vi "chart_clustered.vi"() -> ()   [LabVIEW 8.6]
uses:
  Controls/lxw_chart_type.ctl
  Controls/style_id.ctl
  Controls/lxw_chart_legend_position.ctl
panel:
  out "error out":errorcluster
  out "function return 2":string
  # "chart_clustered2.xlsx"
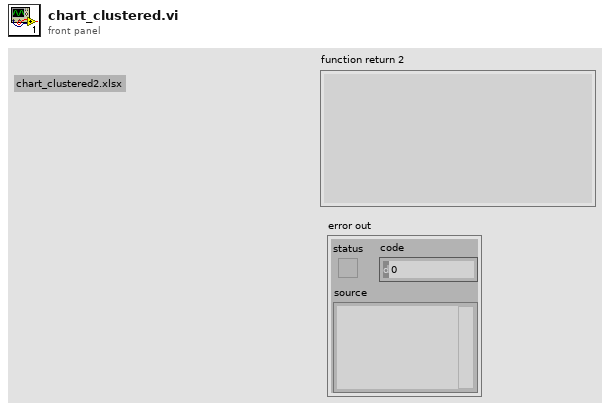
[diagram p1: front panel]
types:
  T1 = typedef "lxw_chart_legend_position.ctl" = u8
  T2 = typedef "style_id.ctl" = u16
  T3 = typedef "lxw_chart_type.ctl" = u8
  T4 = enum32{"invalid app kind", "Development System", "Run Time System", "Student Edition", "Embedded LabVIEW", "Evaluation", "Custom"}
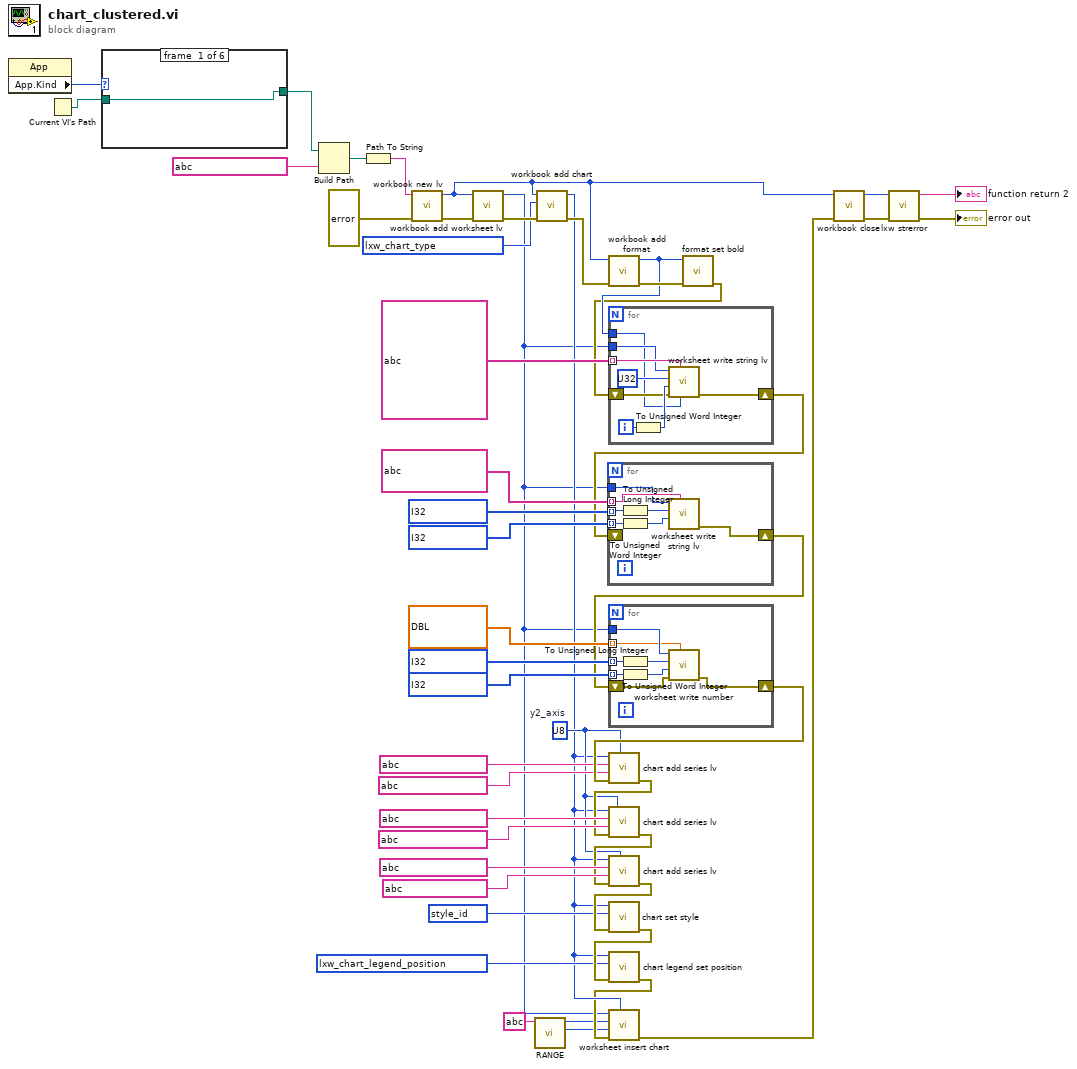
[diagram p0: block diagram]
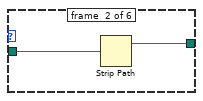
[diagram p2: hidden frame]
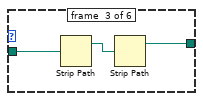
[diagram p3: hidden frame]
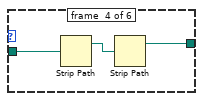
[diagram p4: hidden frame]
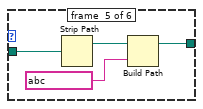
[diagram p5: hidden frame]
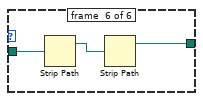
[diagram p6: hidden frame]
diagram:
  w9 = T1 ? items=["LXW_CHART_LEGEND_NONE", "LXW_CHART_LEGEND_RIGHT", "LXW_CHART_LEGEND_LEFT", "LXW_CHART_LEGEND_TOP", "LXW_CHART_LEGEND_BOTTOM", "LXW_CHART_LEGEND_TOP_RIGHT", "LXW_CHART_LEGEND_OVERLAY_RIGHT", "LXW_CHART_LEGEND_OVERLAY_LEFT", "LXW_CHART_LEGEND_OVERLAY_TOP_RIGHT"] ("position")
  w11 = T2 ? items=["Style_1", "Style_2", "Style_3", "Style_4", "Style_5", "Style_6", "Style_7", "Style_8", "Style_9", "Style_10", "Style_11", "Style_12", "Style_13", "Style_14", "Style_15", "Style_16", "Style_17", "Style_18", "Style_19", "Style_20", "Style_21", "Style_22", "Style_23", "Style_24", "Style_25", "Style_26", "Style_27", "Style_28", "Style_29", "Style_30", "Style_31", "Style_32", "Style_33", "Style_34", "Style_35", "Style_36", "Style_37", "Style_38", "Style_39", "Style_40", "Style_41", "Style_42", "Style_43", "Style_44", "Style_45", "Style_46", "Style_47", "Style_48"] ("style_id")
  w12 = u8 ?  # y2_axis
  w27 = T3 ? items=["LXW_CHART_NONE", "LXW_CHART_AREA", "LXW_CHART_AREA_STACKED", "LXW_CHART_AREA_STACKED_PERCENT", "LXW_CHART_BAR", "LXW_CHART_BAR_STACKED", "LXW_CHART_BAR_STACKED_PERCENT", "LXW_CHART_COLUMN", "LXW_CHART_COLUMN_STACKED", "LXW_CHART_COLUMN_STACKED_PERCENT", "LXW_CHART_DOUGHNUT", "LXW_CHART_LINE", "LXW_CHART_LINE_STACKED", "LXW_CHART_LINE_STACKED_PERCENT", "LXW_CHART_PIE", "LXW_CHART_SCATTER", "LXW_CHART_SCATTER_STRAIGHT", "LXW_CHART_SCATTER_STRAIGHT_WITH_MARKERS", "LXW_CHART_SCATTER_SMOOTH", "LXW_CHART_SCATTER_SMOOTH_WITH_MARKERS", "LXW_CHART_RADAR", "LXW_CHART_RADAR_WITH_MARKERS", "LXW_CHART_RADAR_FILLED", "LXW_CHART_STOCK"] ("chart_type")
  n1 = property class="App"() -> ("App.Kind"=w49:T4)  [unwired: 2 in, 2 out]
  n2 = Current VI's Path() -> (path=w48:path)
  n3 = case shown="\"Evaluation\"" w49 {
    tunnel: w48 -> [w50 w52 w55 w58 w62 w65]
    tunnel: [w50 w51 w53 w56 w60 w63] -> w47
    frame #0 {
    }
    frame #1 {
      n4 = Strip Path(path=w52) -> (stripped path=w51:path)  [unwired: 1 out]
    }
    frame #2 {
      n5 = Strip Path(path=w55) -> (stripped path=w54:path)  [unwired: 1 out]
      n6 = Strip Path(path=w54) -> (stripped path=w53:path)  [unwired: 1 out]
    }
    frame #3 {
      n7 = Strip Path(path=w58) -> (stripped path=w57:path)  [unwired: 1 out]
      n8 = Strip Path(path=w57) -> (stripped path=w56:path)  [unwired: 1 out]
    }
    frame #4 {
      n9 = Strip Path(path=w62) -> (stripped path=w61:path)  [unwired: 1 out]
      n10 = Build Path(base path=w61, name or relative path=string ?) -> (appended path=w60:path)
    }
    frame #5 {
      n11 = Strip Path(path=w65) -> (stripped path=w64:path)  [unwired: 1 out]
      n12 = Strip Path(path=w64) -> (stripped path=w63:path)  [unwired: 1 out]
    }
  }
  n13 = Build Path(base path=w47, name or relative path=string ? ("filename")) -> (appended path=w39:path)
  n14 = Path To String(path=w39) -> (string=w38:string)
  n15 = call "workbook new lv.vi"("error in (no error)"=errorcluster ?, "filename"=w38) -> ("error out"=w45:errorcluster, "function return"=w1:u32)  [unwired: 8 in]
  n16 = call "workbook add worksheet lv.vi"("error in (no error)"=w45, "workbook"=w1) -> ("error out"=w28:errorcluster, "function return"=w6:u32)  [unwired: 8 in]
  n17 = call "RANGE.vi"("range_str"=string ?) -> ("col"=w5:u16, "row"=w4:u32)  [unwired: 6 in, 3 out]
  n18 = call "workbook add chart.vi"("error in (no error)"=w28, "chart_type"=w27, "workbook"=w1) -> ("error out"=w26:errorcluster, "function return"=w8:u32)  [unwired: 7 in]
  n19 = call "workbook add format.vi"("error in (no error)"=w26, "workbook"=w1) -> ("error out"=w30:errorcluster, "function return"=w29:u32)  [unwired: 8 in]
  n20 = call "format set bold.vi"("error in (no error)"=w30, "format"=w29) -> ("error out"=w25:errorcluster)  [unwired: 9 in]
  n21 = for {
    tunnel: string[] ? -> [w73] mode=indexing
    tunnel: w6 -> [w72]
    shift-right: [w68] -> w24
    shift-left: w25 -> [w67]
    tunnel: w29 -> [w66]
    i -> [w70]
    n22 = To Unsigned Word Integer(number=w70) -> (unsigned 16bit integer=w69:u16)
    n23 = call "worksheet write string lv.vi"("format"=w66, "string"=w73, "error in (no error)"=w67, "col"=w69, "row"=u32 ?, "worksheet"=w72) -> ("error out"=w68:errorcluster)  [unwired: 4 in, 1 out]
  }
  n24 = for {
    tunnel: string[] ? -> [w80] mode=indexing
    tunnel: i32[] ? -> [w79] mode=indexing
    tunnel: i32[] ? -> [w78] mode=indexing
    tunnel: w6 -> [w77]
    shift-right: [w74] -> w23
    shift-left: w24 -> [_]
    n25 = To Unsigned Long Integer(number=w79) -> (unsigned 32bit integer=w75:u32)
    n26 = To Unsigned Word Integer(number=w78) -> (unsigned 16bit integer=w76:u16)
    n27 = call "worksheet write string lv.vi"("string"=w80, "col"=w76, "row"=w75, "worksheet"=w77) -> ("error out"=w74:errorcluster)  [unwired: 6 in, 1 out]
  }
  n28 = for {
    tunnel: dbl[] ? -> [w83] mode=indexing
    tunnel: i32[] ? -> [w88] mode=indexing
    tunnel: i32[] ? -> [w87] mode=indexing
    tunnel: w6 -> [w86]
    shift-right: [w81] -> w22
    shift-left: w23 -> [w82]
    n29 = To Unsigned Long Integer(number=w88) -> (unsigned 32bit integer=w84:u32)
    n30 = To Unsigned Word Integer(number=w87) -> (unsigned 16bit integer=w85:u16)
    n31 = call "worksheet write number.vi"("number"=w83, "error in (no error)"=w82, "col"=w85, "row"=w84, "worksheet"=w86) -> ("error out"=w81:errorcluster)  [unwired: 5 in, 1 out]
  }
  n32 = call "chart add series lv.vi"("y2_axis"=w12, "error in (no error)"=w22, "values"=string ?, "categories"=string ?, "chart"=w8) -> ("error out"=w17:errorcluster)  [unwired: 5 in, 1 out]
  n33 = call "chart add series lv.vi"("y2_axis"=w12, "error in (no error)"=w17, "values"=string ?, "categories"=string ?, "chart"=w8) -> ("error out"=w14:errorcluster)  [unwired: 5 in, 1 out]
  n34 = call "chart add series lv.vi"("y2_axis"=w12, "error in (no error)"=w14, "values"=string ?, "categories"=string ?, "chart"=w8) -> ("error out"=w13:errorcluster)  [unwired: 5 in, 1 out]
  n35 = call "chart set style.vi"("error in (no error)"=w13, "style_id"=w11, "chart"=w8) -> ("error out"=w10:errorcluster)  [unwired: 8 in]
  n36 = call "chart legend set position.vi"("error in (no error)"=w10, "position"=w9, "chart"=w8) -> ("error out"=w7:errorcluster)  [unwired: 8 in]
  n37 = call "worksheet insert chart.vi"("chart"=w8, "error in (no error)"=w7, "col"=w5, "row"=w4, "worksheet"=w6) -> ("error out"=w2:errorcluster)  [unwired: 5 in, 1 out]
  n38 = call "workbook close.vi"("error in (no error)"=w2, "workbook"=w1) -> ("error out"=w41:errorcluster, "function return"=w43:u32)  [unwired: 8 in]
  n39 = call "lxw strerror.vi"("error in (no error)"=w41, "error_num"=w43) -> ("error out"=→"error out":errorcluster, "function return"=→"function return 2":string)  [unwired: 8 in]
